vi "Marshal.vi"(8 "error in (no error)":errorcluster, 11 "int32 in":refnum<class "bytes.lvclass">) -> (0 "error out":errorcluster, 2 "Buffer":u8[](array[numeric]), 3 "int32 out":refnum<class "bytes.lvclass">)   [LabVIEW 2020, in "Protobuf RAW.lvlib" / "bytes.lvclass"]
uses:
  bytes.lvclass
  bytes.lvclass/bytes.ctl
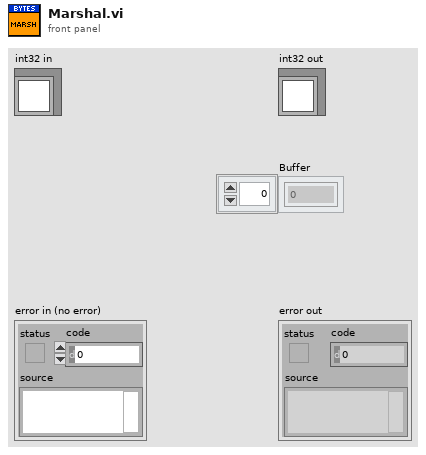
[diagram p1: front panel]
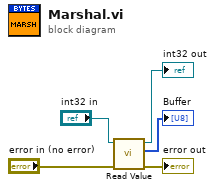
[diagram p0: block diagram]
diagram:
  n1 = call "Read Value.vi"("error in (no error)"="error in (no error)", "fixed32 in"="int32 in") -> ("error out"=→"error out":errorcluster, "Value"=→"Buffer":u8[], "fixed32 out"=→"int32 out":refnum<class "bytes.lvclass">)  [unwired: 7 in]
